vi "Create from Element.vi"(8 "error in (no error)":errorcluster, 10 "Config Element":refnum<class "Config Element.lvclass">, 11 "Seq Element in":refnum<class "Seq Element.lvclass">) -> (0 "error out":errorcluster, 3 "Seq Element out":refnum<class "Seq Element.lvclass">)   [LabVIEW 2020, in "Seq Element.lvclass"]
uses:
  Seq Element.lvclass
  lv-cdm/CDM-Config/Config Element/Config Element.lvclass
  Seq Element.lvclass/Seq Element.ctl
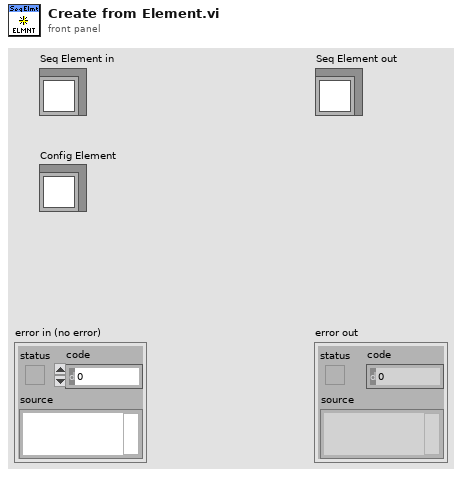
[diagram p1: front panel]
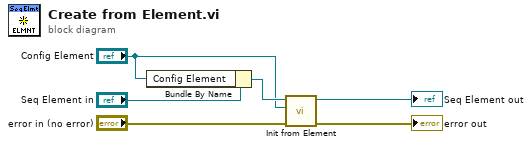
[diagram p0: block diagram]
diagram:
  n1 = Bundle By Name(cluster="Seq Element in", "Config Element"="Config Element") -> (w4:refnum<class "Seq Element.lvclass">)
  n2 = call-dynamic "Init from Element.vi"("error in (no error)"="error in (no error)", "Config Element"="Config Element", "Seq Element in"=w4) -> ("error out"=→"error out":errorcluster, "Seq Element out"=→"Seq Element out":refnum<class "Seq Element.lvclass">)  [unwired: 7 in]
